vi "BotSpeak_Stepper.vi"(2 "DIO Line":u8(slide) scale=0.0..3.0, 3 "# pulses":u32=2, 4 "Bot Settings":T1) -> (0 "response":string="169.254.32.85", 1 "Bot Settings 2":T1)   [LabVIEW 2012]
doc: "Drives a stepper motor via the RIO. Given the \"DIO line\" to which the stepper is wired, the stepper will turn the specified \"number of pulses\"."
uses:
  <userlib>/BotSpeak/VIs/Direct/BotSpeak_Control.ctl
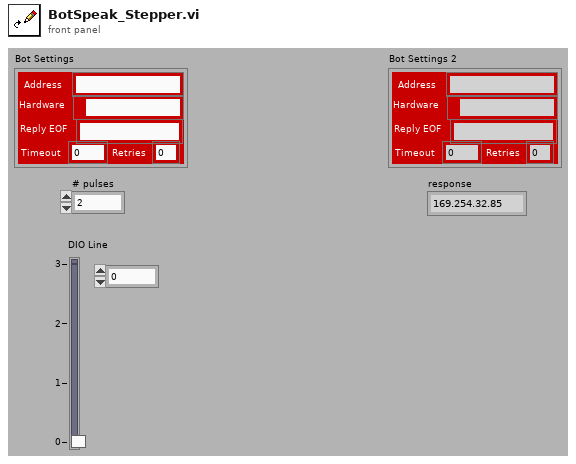
[diagram p1: front panel]
types:
  T1 = typedef "BotSpeak_Control.ctl" = cluster{"Address":string, "Reply EOF":string, "Hardware":path, "Retries":i8, "Timeout":i32}
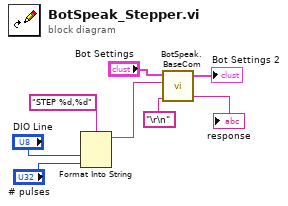
[diagram p0: block diagram]
diagram:
  n1 = Format Into String(format string="STEP %d,%d" ("command"), "DIO Line", "# pulses") -> (resulting string=w2:string)  [unwired: 2 in, 1 out]
  n2 = call <userlib>:"BotSpeak.BaseCom.vi"("Termination"="\r\n", "command"=w2, "Bot Settings in"="Bot Settings") -> ("response"=→"response":string, "Bot Settings out"=→"Bot Settings 2":T1)  [unwired: 2 in]
